vi "CullandGroupGear.vi"(6 "Line Border":cluster{"Top":dbl, "Bottom":dbl}={"Top"=6.0, "Bottom"=1.0}, 9 "Score Cutoff":dbl=3.0, 10 "Sorted Data":dbl[][](array[numeric])) -> (0 "Rect":T1, 1 "Line":T1, 2 "Score":dbl, 3 "Center":cluster{"X":dbl, "Y":dbl})   [LabVIEW 2016]
doc: "Examine the particle measurements to find the most likely pair that make up the target. This mostly compares the edges of the bounding boxes. It then returns information about the overall target, notably the rectangle sourrounding the particles, the vertical line that bisects the target, and the center of the top particle."
panel:
  out "Grouping Scores":T2(array[cluster])
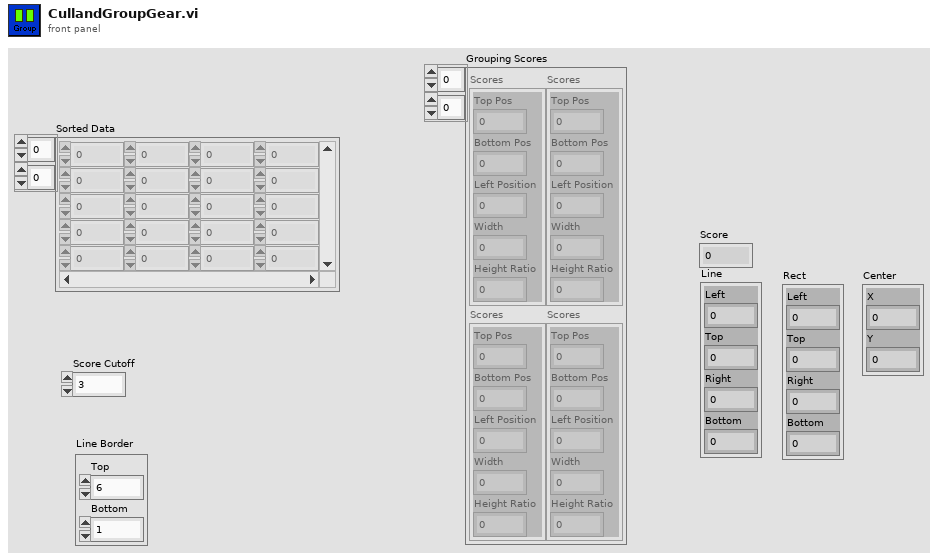
[diagram p1: front panel]
types:
  T1 = cluster{"Left":dbl, "Top":dbl, "Right":dbl, "Bottom":dbl}
  T2 = cluster{"Top Pos":dbl, "Bottom Pos":dbl, "Left Position":dbl, "Width":dbl, "Height Ratio":dbl}[][]
  T3 = cluster{"Top Position":dbl, "Bottom Position":dbl, "Left Gap":dbl, "Width":dbl, "Height Ratio":dbl}
  T4 = cluster{"Left":dbl, "Numeric":dbl, "Right":dbl, "Numeric":dbl}
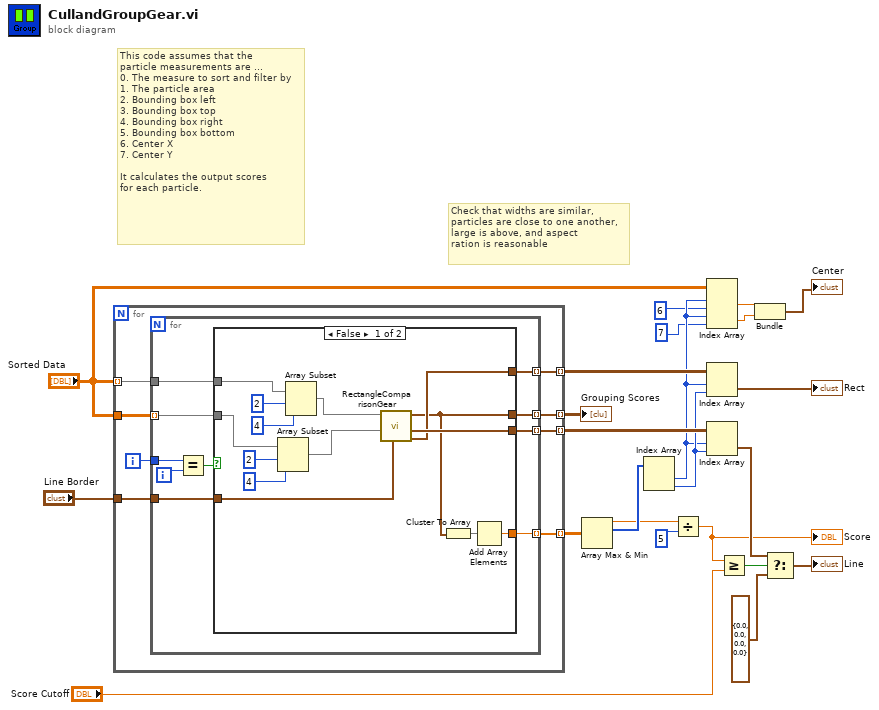
[diagram p0: block diagram]
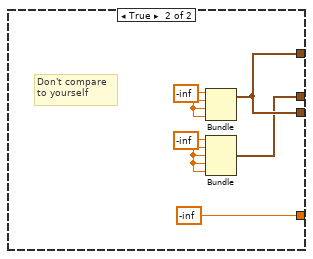
[diagram p2: hidden frame]
diagram:
  # "Check that widths are similar,\nparticles are close to one another,\nlarge is above, and aspect\nration is reasonable"
  # "This code assumes that the\nparticle measurements are ...\n0. The measure to sort and filter by\n1. The particle area\n2. Bounding box left\n3. Bounding box top\n4. Bounding box right\n5. Bounding box bottom\n6. Center X\n7. Center Y\n\nIt calculates the output scores\nfor each particle."
  n1 = for {
    tunnel: "Sorted Data" -> [w31] mode=indexing
    tunnel: "Sorted Data" -> [w30]
    tunnel: [w29] -> w23 mode=indexing
    tunnel: [w27] -> w22 mode=indexing
    tunnel: [w26] -> w19 mode=indexing
    tunnel: [w25] -> w15 mode=indexing
    tunnel: "Line Border" -> [w24]
    i -> [w28]
    n2 = for {
      tunnel: w31 -> [w41]
      tunnel: w30 -> [w39] mode=indexing
      tunnel: [w38] -> w29 mode=indexing
      tunnel: w28 -> [w37]
      tunnel: [w35] -> w27 mode=indexing
      tunnel: [w34] -> w26 mode=indexing
      tunnel: [w33] -> w25 mode=indexing
      tunnel: w24 -> [w32]
      i -> [w36]
      n3 = Equal?(x=w37, y=w36) -> (x = y?=w40:bool)
      n4 = case shown="False" w40 {
        tunnel: w41 -> [w53 _]
        tunnel: w39 -> [w50 _]
        tunnel: [w45 w56] -> w38
        tunnel: [w48 -inf] -> w35
        tunnel: [w47 w59] -> w34
        tunnel: [w46 w59] -> w33
        tunnel: w32 -> [w44 _]
        frame False {
          n5 = Array Subset(array=w50, index=2, length=4) -> (w42:dbl[])
          n6 = Array Subset(array=w53, index=2, length=4) -> (w43:dbl[])
          n7 = call "RectangleComparisonGear.vi"("Line Border"=w44, "Second"=w42, "First"=w43) -> ("Rect"=w46:T1, "Line"=w47:T1, "Scores"=w45:T3)  [unwired: 6 in]
          n8 = Cluster To Array(cluster=w45) -> (array=w49:dbl[])
          n9 = Add Array Elements(numeric array=w49) -> (sum=w48:dbl)
        }
        frame True {
          w57 = -inf
          w58 = -inf
          # "Don't compare\nto yourself"
          n10 = Bundle(w58, w58, w58, w58) -> (w59:cluster{dbl, dbl, dbl, dbl})  [unwired: 1 in]
          n11 = Bundle(w57, w57, w57, w57, w57) -> (w56:cluster{dbl, dbl, dbl, dbl, dbl})  [unwired: 1 in]
        }
      }
    }
  }
  "Grouping Scores" <- w23
  n12 = Array Max & Min(array=w22) -> (max value=w4:dbl, max index (indices)=w5:i32[])  [unwired: 2 out]
  n13 = Index Array(array=w5) -> (element #1=w11:i32, element #2=w14:i32)  [unwired: 2 in]
  n14 = Divide(x=w4, y=5 ("length")) -> (x/y=w3:dbl)
  "Score" <- w3
  n15 = Index Array(array="Sorted Data", index (row) #1=w11, index (col) #1=6 ("index"), index (row) #2=w11, index (col) #2=7 ("index")) -> (element #1=w9:dbl, element #2=w8:dbl)
  n16 = Index Array(array=w15, index (row)=w11, index (col)=w14) -> (element=→"Rect":T1)
  n17 = Index Array(array=w19, index (row)=w11, index (col)=w14) -> (element=w18:T1)
  n18 = Greater Or Equal?(x=w3, y="Score Cutoff") -> (x >= y?=w21:bool)
  n19 = Bundle("Numeric"=w9, "Numeric"=w8) -> (→"Center":cluster{"Numeric":dbl, "Numeric":dbl})  [unwired: 1 in]
  n20 = Select(t=w18, s=w21, f=cluster{dbl, "Numeric":dbl, dbl, "Numeric":dbl} {0.0, "Numeric"=0.0, 0.0, "Numeric"=0.0}) -> (s? t:f=→"Line":T4)
